vi "Execute Search To Mark.vi"(9 "Plot length scale":dbl format="%#_13g", 10 "Point Phase":dbl[](array[numeric]), 11 "Data [magnitude,Phase]In":cluster{"magnitude 2":dbl, "phase":dbl}[](array[cluster])) -> (3 "Data [magnitude,Phase] Out":cluster{"magnitude 2":dbl, "phase":dbl}[](array[cluster]))   [LabVIEW 2020]
uses:
  ec845b71-826e-4634-98c5-25ffb071b0a3.vi
  <vilib>/Comparison/Equal/Equal Functor/Equal Functor.lvclass
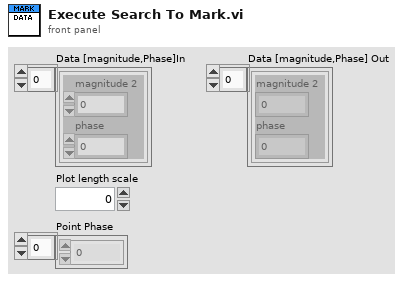
[diagram p1: front panel]
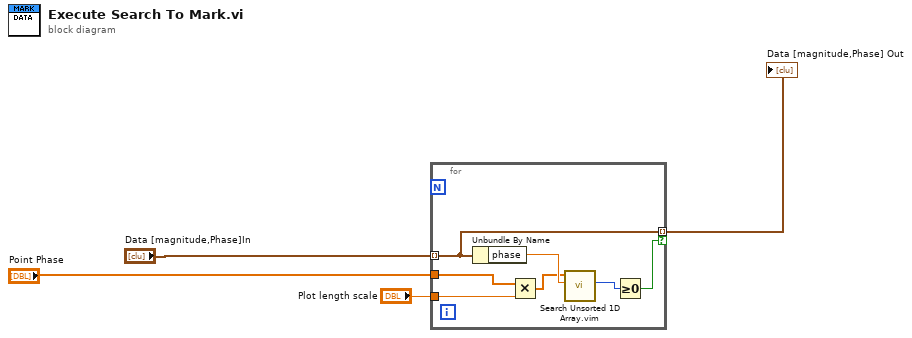
[diagram p0: block diagram]
diagram:
  n1 = for {
    tunnel: "Data [magnitude,Phase]In" -> [w11] mode=indexing
    tunnel: "Point Phase" -> [w6]
    tunnel: [w11] -> w4 mode=indexing if=w9
    tunnel: "Plot length scale" -> [w8]
    n2 = Unbundle By Name(w11) -> ("phase"=w7:dbl)
    n3 = Multiply(x=w6, y=w8) -> (x*y=w5:dbl[])
    n4 = call "Search Unsorted 1D Array.vim"("element"=w7, "unsorted 1D array"=w5) -> ("index of element"=w10:i32)  [unwired: 9 in]
    n5 = Greater Or Equal To 0?(x=w10) -> (x >= 0?=w9:bool)
  }
  "Data [magnitude,Phase] Out" <- w4
